vi "ep_Scale FFT Array for RMS.vi"(10 "f0":dbl format="%.2f", 11 "FFT{X} [EU]":cdb[](array[numeric]) format="%.2f") -> (3 "FFT {X} [rms]":cdb[](array[numeric]) format="%.2f")   [LabVIEW 2014, in "NI_EP_Motor Monitoring.lvlib"]
uses:
  <vilib>/addons/Electrical Power/Motor Monitoring/NI_EP_Motor Monitoring.lvlib
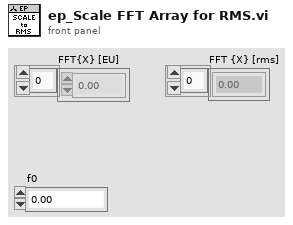
[diagram p1: front panel]
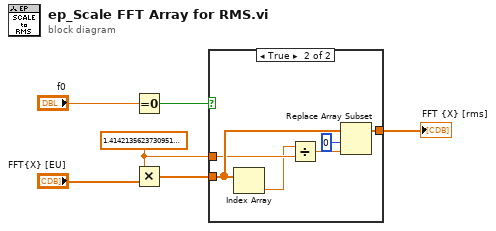
[diagram p0: block diagram]
diagram:
  w5 = cdb 1.4142135623730951+0.0i ("sqrt(x)")
  n1 = Equal To 0?(x="f0") -> (x = 0?=w1:bool)
  n2 = Multiply(x=w5, y="FFT{X} [EU]") -> (x*y=w3:cdb[])
  n3 = case shown="True" w1 {
    tunnel: w3 -> [w7 w11]
    tunnel: w5 -> [_ w10]
    tunnel: [w7 w8] -> w2
    frame False {
    }
    frame True {
      n4 = Index Array(array=w11) -> (element=w9:cdb)  [unwired: 1 in]
      n5 = Divide(x=w9, y=w10) -> (x/y=w12:cdb)
      n6 = Replace Array Subset(array=w11, new element=w12, index=0 ("Index")) -> (w8:cdb[])
    }
  }
  "FFT {X} [rms]" <- w2
